vi "Handle Message.vi"(0 "ICanCommunicate In":refnum<class "ICanCommunicate.lvclass">, 7 "Message In":T1, 11 "Error In":errorcluster) -> (4 "ICanCommunicate Out":refnum<class "ICanCommunicate.lvclass">, 6 "CMD Out":string, 8 "Message Out":T1, 15 "Error Out":errorcluster)   [LabVIEW 2023, in "ICanCommunicate.lvclass"]
doc: "Specifies the way of handling incoming messages."
uses:
  ICanCommunicate.lvclass
  Message.ctl
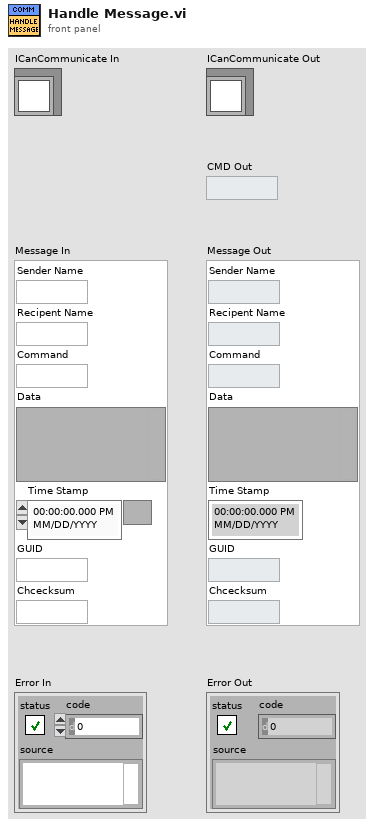
[diagram p1: front panel]
types:
  T1 = typedef "ICanCommunicate.lvclass/Message.ctl" = cluster{"Sender Name":string, "Recipent Name":string, "Command":string, "Data":variant, "Time Stamp":timestamp, "GUID":string, "Chcecksum":string}
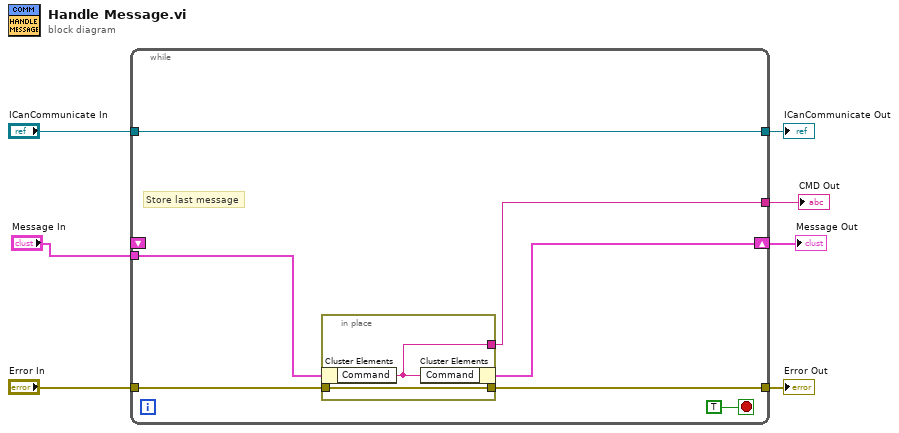
[diagram p0: block diagram]
diagram:
  n1 = while {
    shift-right: [w10] -> w3
    shift-left: _ -> [_]
    tunnel: "Error In" -> [w12]
    tunnel: [w11] -> w6
    tunnel: "ICanCommunicate In" -> [w14]
    tunnel: [w14] -> w4
    tunnel: "Message In" -> [w8]
    tunnel: [w9] -> w1
    stop <- TRUE stop-if-true
    # "Store last message"
    n2 = in-place {
      in-place-border: [w15] -> w9
      in-place-border: [w16] -> w11
      in-place-border: w12 -> [w16]
      n3 = in-place-cluster #1(w8) -> ("Command"=w15:string)
      n4 = in-place-cluster #1("Command"=w15) -> (w10:T1)
    }
  }
  "Error Out" <- w6
  "ICanCommunicate Out" <- w4
  "Message Out" <- w3
  "CMD Out" <- w1
